vi "LaneFollow.vi"(3 "SupressIn":dbl, 7 "Inhibit":bool, 8 "HowAmI? Clean":cluster{"T":dbl, "Battery":dbl, "Temp":dbl}, 9 "WhatAroundMe? Clean":cluster{"T":dbl, "Range":dbl, "Bearing":dbl}[](array[cluster]), 10 "WhereAmI? Clean":T1, 11 "Velocity":dbl) -> (0 "SupressOut":dbl, 2 "ActCommand":dbl[](array[numeric]), 4 "InhibitOut":bool)   [LabVIEW 2012]
doc: "This subVI executes alane folowing Midbrain behaviors. Its inputs are the outputs of the three SENSE processes, the overall velocity requested of the robot, a suppression value from another co-brahvior and an inhibit signal to turn the behavior off. The outputs are a 90 element steering array, a suppression value to diminish the output of co-behaviors and an inhibit output to shut off otehr behaviors.\n\nIt is designed to work with a 90 element behavior arbiter."
uses:
  <vilib>/Analysis/2dsp.llb/Integral Method.ctl
  <vilib>/Analysis/1siggen.llb/Ramp Pattern by Samples.vi
  <vilib>/Analysis/8numeric.llb/1D Numeric Integration.vi
  <vilib>/gmath/statdist.llb/Normal PDF.vi
  <vilib>/Analysis/NI_AALPro.lvlib
  <vilib>/gmath/NI_Gmath.lvlib
  <vilib>/Analysis/NI_AALBase.lvlib
panel:
  out "LaneGain":dbl
  out "std (Normal)":dbl
  out "Waveform Graph":dbl[][](graph)
  out "x+y":dbl
  # "This VI contains a lane following behavior at the Midbrain level"
  # "0.8"
  # "2"
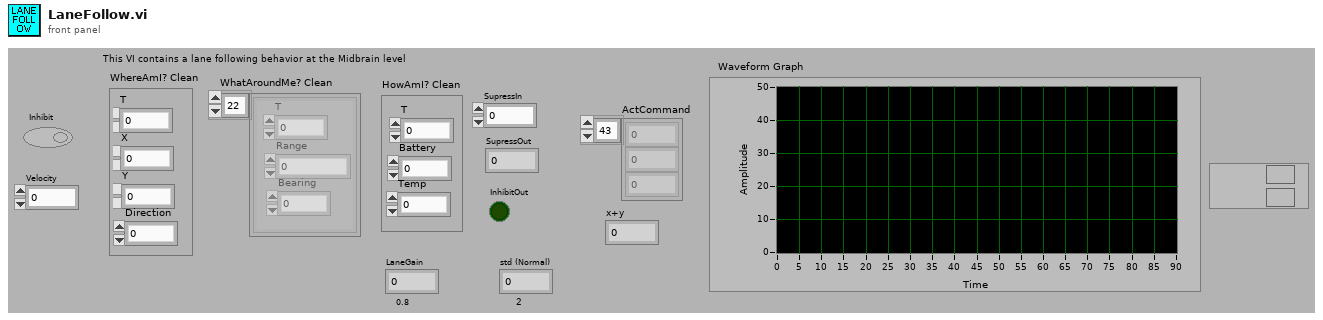
[diagram p1: front panel]
types:
  T1 = cluster{"T":dbl, "X":dbl, "Y":dbl, "Direction":dbl}
  T2 = typedef "NI_AALPro.lvlib/Integral Method.ctl" = i32
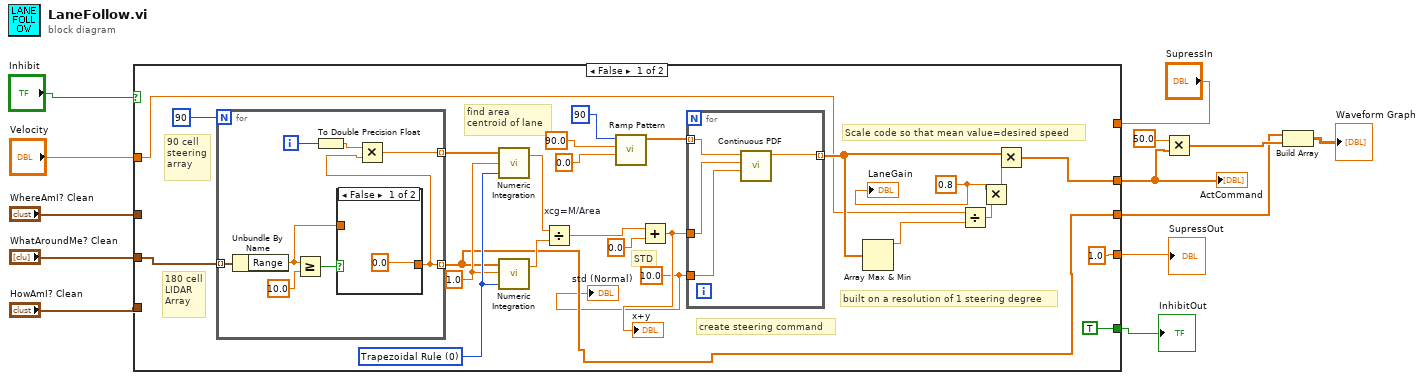
[diagram p0: block diagram]
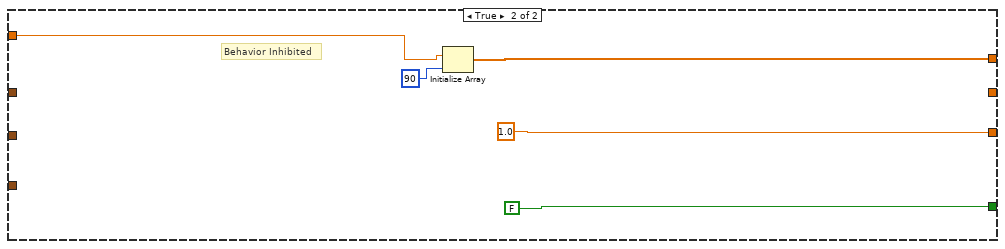
[diagram p3: hidden frame]
diagram:
  n1 = case shown="False" "Inhibit" {
    tunnel: "Velocity" -> [w16 w53]
    tunnel: "WhatAroundMe? Clean" -> [w19 _]
    tunnel: "WhereAmI? Clean" -> [_ _]
    tunnel: "HowAmI? Clean" -> [_ _]
    tunnel: "SupressIn" -> [_ _]
    tunnel: [w18 w55] -> w3
    tunnel: [1.0 ("SupressOut") 1.0 ("SupressOut")] -> w7
    tunnel: [TRUE ("InhibitOut") FALSE ("InhibitOut")] -> w6
    tunnel: [w17 _] -> w1
    frame False {
      w15 = 10.0 ("std (Normal)")
      w14 = 0.8 ("x")
      w22 = 1.0 ("dt")
      w23 = T2 0 items=["Trapezoidal Rule", "Simpson's Rule", "Simpson's 3/8 Rule", "Bode Rule"] ("integration method")
      # "create steering command"
      # "find area\ncentroid of lane"
      # "built on a resolution of 1 steering degree"
      # "Scale code so that mean value=desired speed"
      # "STD"
      # "180 cell\nLIDAR \nArray"
      # "90 cell\nsteering\narray"
      n2 = for {
        N: 90 -> [_]
        tunnel: w19 -> [w50] mode=indexing
        tunnel: [w45] -> w17 mode=indexing
        tunnel: [w43] -> w21 mode=indexing
        i -> [w46]
        n3 = Unbundle By Name(w50) -> ("Range"=w47:dbl)
        n4 = Greater Or Equal?(x=w47, y=10.0) -> (x >= y?=w48:bool)
        n5 = To Double Precision Float(number=w46) -> (double precision float=w44:dbl)
        n6 = case shown="False" w48 {
          tunnel: w47 -> [_ w52]
          tunnel: [0.0 ("Range") w52] -> w45
          frame False {
          }
          frame True {
          }
        }
        n7 = Multiply(x=w44, y=w45) -> (x*y=w43:dbl)
      }
      n8 = call-poly <vilib>:"Numeric Integration.vi"("integration method"=w23, "dt"=w22, "Input Array"=w21) -> ("result"=w31:dbl)  [unwired: 1 out]
      n9 = call-poly <vilib>:"Numeric Integration.vi"("integration method"=w23, "dt"=w22, "Input Array"=w17) -> ("result"=w24:dbl)  [unwired: 1 out]
      n10 = Divide "xcg=M/Area"(x=w31, y=w24) -> (x/y=w32:dbl)
      n11 = call-poly <vilib>:"Ramp Pattern.vi"("start"=0.0, "end"=90.0 ("end (Normal)"), "samples"=90) -> ("Ramp Pattern"=w35:dbl[])  [unwired: 7 in, 1 out]
      n12 = Add(x=w32, y=0.0) -> (x+y=w33:dbl)
      "x+y" <- w33
      n13 = for {
        tunnel: w35 -> [w42] mode=indexing
        tunnel: w15 -> [w41]
        tunnel: [w40] -> w25 mode=indexing
        tunnel: w33 -> [w39]
        n14 = call-poly <vilib>:"Continuous PDF.vi"("std"=w41, "mean"=w39, "x"=w42) -> ("pdf(x)"=w40:dbl)  [unwired: 7 in, 1 out]
      }
      n15 = Array Max & Min(array=w25) -> (max value=w27:dbl)  [unwired: 3 out]
      n16 = Divide(x=w16, y=w27) -> (x/y=w26:dbl)
      n17 = Multiply(x=w14, y=w26) -> (x*y=w36:dbl)
      n18 = Multiply(x=w25, y=w36) -> (x*y=w18:dbl[])
      "std (Normal)" <- w15
      "LaneGain" <- w14
    }
    frame True {
      # "Behavior Inhibited"
      n19 = Initialize Array "Initialize Array"(w53, 90 ("dimension size")) -> (w55:dbl[])
    }
  }
  "ActCommand" <- w3
  "SupressOut" <- w7
  "InhibitOut" <- w6
  n20 = Multiply(x=50.0, y=w3) -> (x*y=w2:dbl[])
  n21 = Build Array(w1, w2) -> (→"Waveform Graph":dbl[][])
